vi "Write Hardware Handles.vi"(8 "error in":errorcluster, 10 "hardware handles":T1, 11 "AIM ARINC-429 shared resources in":refnum<class "Shared Resources.lvclass">) -> (0 "error out":errorcluster, 3 "AIM ARINC-429 shared resources out":refnum<class "Shared Resources.lvclass">)   [LabVIEW 2020, in "AIM ARINC 429 Engine.lvlib" / "Implementation.lvlib" / "Shared Resources.lvclass"]
uses:
  Shared Resources.lvclass
  Custom Device/Hardware Handles.ctl
  Custom Device/Custom Device.lvlib
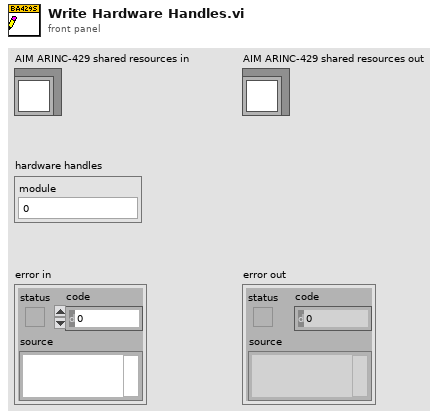
[diagram p1: front panel]
types:
  T1 = typedef "AIM ARINC 429 Engine.lvlib/Custom Device.lvlib/Hardware Handles.ctl" = cluster{"module":u8}
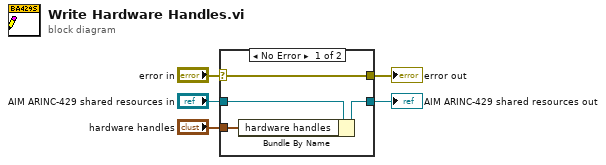
[diagram p0: block diagram]
diagram:
  n1 = case shown="No Error" "error in" {
    selector: "error in" -> [w9 w10]
    tunnel: [w9 w10] -> w4
    tunnel: [w6 w11] -> w2
    tunnel: "AIM ARINC-429 shared resources in" -> [w8 w11]
    tunnel: "hardware handles" -> [w7 _]
    frame No Error {
      n2 = Bundle By Name(cluster=w8, "hardware handles"=w7) -> (w6:refnum<class "Shared Resources.lvclass">)
    }
    frame Error {
    }
  }
  "error out" <- w4
  "AIM ARINC-429 shared resources out" <- w2
